vi "Subset.vi"(7 "length (-1: rest)":i64=-1 format="%d bytes", 8 "error in (no error)":errorcluster, 9 "offset (0)":u64 format="%d bytes", 10 "subset Pointer type":refnum<class "Pointer.lvclass">, 11 "base Pointer in":refnum<class "Pointer.lvclass">) -> (0 "error out":errorcluster, 1 "offset + size":u64 format="%d bytes", 2 "subset Pointer":refnum<class "Pointer.lvclass">, 3 "base Pointer out":refnum<class "Pointer.lvclass">)   [LabVIEW 2027, in "Memory Manager.lvlib" / "Pointer.lvclass"]
doc: "Creates a new <b>subset Pointer</b> object that represents a subset of the provided <b>base Pointer</b> block."
uses:
  Pointer.lvclass
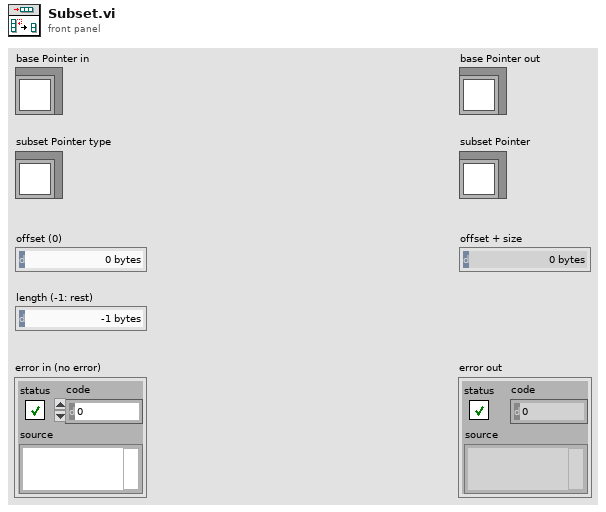
[diagram p1: front panel]
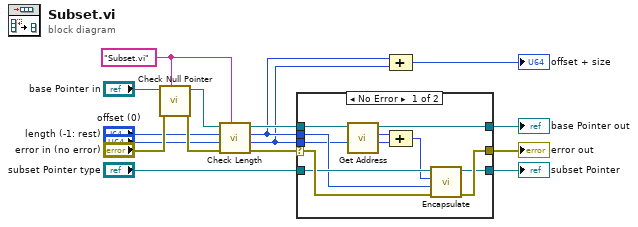
[diagram p0: block diagram]
diagram:
  w13 = "Subset.vi" ("source vi name")
  n1 = call "Check Null Pointer.vi"("source vi name"=w13, "error in (no error)"="error in (no error)", "Pointer in"="base Pointer in") -> ("error out"=w6:errorcluster, "Pointer out"=w11:refnum<class "Pointer.lvclass">)  [unwired: 7 in]
  n2 = call "Check Length.vi"("source vi name"=w13, "error in (no error)"=w6, "offset (0)"="offset (0)", "length (-1: rest)"="length (-1: rest)", "Pointer in"=w11) -> ("error out"=w9:errorcluster, "offset"=w3:u64, "size"=w4:u64, "Pointer out"=w10:refnum<class "Pointer.lvclass">)  [unwired: 3 in]
  n3 = case shown="No Error" w9 {
    selector: w9 -> [w26 w27]
    tunnel: "subset Pointer type" -> [w25 w28]
    tunnel: [w23 w28] -> w15
    tunnel: w10 -> [w22 w29]
    tunnel: [w21 w29] -> w14
    tunnel: w4 -> [w18 _]
    tunnel: w3 -> [w17 _]
    tunnel: [w24 w27] -> w12
    frame No Error {
      n4 = call "Get Address.vi"("Pointer in"=w22) -> ("address"=w20:u64, "Pointer out"=w21:refnum<class "Pointer.lvclass">)  [unwired: 9 in]
      n5 = Compound Arithmetic op=ADD(w20, w17) -> (w19:u64)
      n6 = call "Encapsulate.vi"("error in (no error)"=w26, "size"=w18, "address"=w19, "Pointer type"=w25) -> ("error out"=w24:errorcluster, "Pointer"=w23:refnum<class "Pointer.lvclass">)  [unwired: 6 in]
    }
    frame Error {
    }
  }
  "error out" <- w12
  "subset Pointer" <- w15
  "base Pointer out" <- w14
  n7 = Compound Arithmetic op=ADD(w4, w3) -> (→"offset + size":u64)
